vi "log analysis_gps.vi"() -> ()   [LabVIEW 2018] (continued)
status\t114.221582\t125.488390\t7.927600\t-0.997618\t-0.087714\t0.790594\t0.306000\t-0.022000\n\t\n15:12:16.9\tlog_raw\tgps_raw\t\tsystem status\tnormal 2 28.000000 0 0\trobot status\t114.369285\t125.472789\t7.927800\t-0.675524\t-0.152643\t0.044977\t0.313000\t0.000000\n\t\n15:12:17.4\tlog_raw\tgps_raw\t\tsystem status\tnormal 2 28.100000 0 0\trobot status\t114.509051\t125.458503\t7.927000\t-0.401404\t-0.017931\t-0.437891\t0.274000\t-0.037000\n\t\n15:12:17.9\tlog_raw\tgps_raw\t\tsystem status\tnormal 2 28.200000 0 0\trobot status\t114.650658\t125.444370\t7.924700\t-0.327337\t-0.035716\t-0.663327\t0.335000\t0.061000\n\t\n15:12:18.4\tlog_raw\tgps_raw\t\tsystem status\tnormal 2 28.200000 0 0\trobot status\t114.786676\t125.428978\t7.924000\t-0.306443\t0.009430\t-0.778391\t0.296000\t0.002000\n\t\n15:12:18.9\tlog_raw\tgps_raw\t\tsystem status\tnormal 2 28.200000 0 0\trobot status\t114.917132\t125.412522\t7.923700\t-0.381803\t-0.145453\t-0.928746\t0.292000\t0.032000\n\t\n15:12:19.4\tlog_raw\tgps_raw\t#INSPVAXA,USB3,0,47.5,FINESTEERING,2107,281557.450,02000000,471d,15824;INS_ALIGNMENT_COMPLETE,INS_RTKFIXED,37.37126007127,126.72213399175,7.9228,22.3000,-0.0436,0.2932,0.0085,-0.364989974,-0.412142636,90.870623018,0.4100,0.2787,0.5090,0.1093,0.0914,0.0751,0.1708,0.1703,5.1179,0f000001,0*5c4f0bd9\n\tsystem status\tnormal 2 28.200000 0 0\trobot status\t115.053253\t125.397910\t7.922800\t-0.364990\t-0.412143\t-0.870623\t0.296000\t0.029000\n\t\n15:12:19.9\tlog_raw\tgps_raw\t\tsystem status\tnormal 2 28.200000 0 0\trobot status\t115.206485\t125.383092\t7.922200\t-0.467906\t-0.695573\t-0.896423\t0.313000\t0.011000\n\t\n15:12:20.4\tlog_raw\tgps_raw\t#INSPVAXA,USB3,0,46.0,FINESTEERING,2107,281558.450,02000000,471d,15824;INS_ALIGNMENT_COMPLETE,INS_RTKFIXED,37.37125980811,126.72213741354,7.9201,22.3000,-0.0396,0.2827,0.0144,-0.665732137,-0.749833579,90.834139291,0.4087,0.2784,0.5089,0.1102,0.0917,0.0750,0.1706,0.1703,5.1108,0f000001,0*c48606ec\n\tsystem status\tnormal 2 28.200000 0 0\trobot status\t115.356349\t125.368699\t7.920100\t-0.665732\t-0.749834\t-0.834139\t0.304000\t0.025000\n\t\n15:12:20.9\tlog_raw\tgps_raw\t#INSPVAXA,USB3,0,46.0,FINESTEERING,2107,281558.950,02000000,471d,15824;INS_ALIGNMENT_COMPLETE,INS_RTKFIXED,37.37125968631,126.72213896635,7.9182,22.3000,-0.0389,0.2938,0.0155,-0.920394419,-0.718289974,90.450245046,0.4087,0.2784,0.5089,0.1102,0.0917,0.0750,0.1706,0.1703,5.1108,0f000001,0*246e9289\n\tsystem status\tnormal 2 28.100000 0 0\trobot status\t115.493895\t125.355179\t7.918200\t-0.920394\t-0.718290\t-0.450245\t0.249000\t0.114000\n\t\n15:12:21.4\tlog_raw\tgps_raw\t\tsystem status\tnormal 2 28.000000 0 0\trobot status\t115.630698\t125.346330\t7.917200\t-1.162131\t-0.468007\t0.253588\t0.446000\t-0.179000\n\t\n15:12:21.9\tlog_raw\tgps_raw\t\tsystem status\tnormal 2 27.800000 0 0\trobot status\t115.765858\t125.337595\t7.917100\t-1.166059\t-0.209955\t1.295503\t0.319000\t0.012000\n\t\n15:12:22.4\tlog_raw\tgps_raw\t\tsystem status\tnormal 2 27.900000 0 0\trobot status\t115.901706\t125.332414\t7.918000\t-1.105135\t-0.074497\t2.615411\t0.302000\t0.044000\n\t\n15:12:22.9\tlog_raw\tgps_raw\t\tsystem status\tnormal 2 27.800000 0 0\trobot status\t116.038405\t125.330658\t7.919000\t-1.227928\t0.059274\t3.935949\t0.290000\t0.054000\n\t\n15:12:23.4\tlog_raw\tgps_raw\t\tsystem status\tnormal 2 27.800000 0 0\trobot status\t116.176515\t125.336559\t7.920100\t-1.592116\t0.311870\t5.113002\t0.303000\t0.035000\n\t\n15:12:23.9\tlog_raw\tgps_raw\t\tsystem status\tnormal 2 27.900000 0 0\trobot status\t116.315239\t125.343681\t7.923900\t-1.641729\t0.301308\t6.150827\t0.304000\t0.038000\n\t\n15:12:24.4\tlog_raw\tgps_raw\t\tsystem status\tnormal 2 27.900000 0 0\trobot status\t116.455707\t125.354228\t7.925400\t-1.548111\t0.138625\t6.918070\t0.290000\t0.040000\n\t\n15:12:24.9\tlog_raw\tgps_raw\t\tsystem status\tnormal 2 28.000000 0 0\trobot status\t116.600236\t125.367270\t7.927000\t-1.578539\t-0.051102\t7.497431\t0.293000\t0.033000\n\t\n15:12:25.4\tlog_raw\tgps_raw\t\tsystem status\tnormal 2 28.100000 0 0\trobot status\t116.741361\t125.382496\t7.928200\t-1.712113\t-0.033243\t7.732061\t0.302000\t0.000000\n\t\n15:12:25.9\tlog_raw\tgps_raw\t\tsystem status\tnormal 2 28.100000 0 0\trobot status\t116.883583\t125.398503\t7.929100\t-1.939151\t-0.176263\t7.869611\t0.273000\t0.043000\n\t\n15:12:26.4\tlog_raw\tgps_raw\t\tsystem status\tnormal 2 28.200000 0 0\trobot status\t117.028703\t125.414022\t7.929100\t-2.090861\t-0.326492\t7.769708\t0.280000\t0.022000\n\t\n15:12:26.9\tlog_raw\tgps_raw\t\tsystem status\tnormal 2 28.200000 0 0\trobot status\t117.168081\t125.427820\t7.929300\t-2.230499\t-0.413156\t7.644957\t0.298000\t-0.014000\n\t\n15:12:27.4\tlog_raw\tgps_raw\t\tsystem status\tnormal 2 28.200000 0 0\trobot status\t117.306809\t125.442252\t7.930200\t-2.373589\t-0.461391\t7.481825\t0.295000\t-0.036000\n\t\n15:12:27.9\tlog_raw\tgps_raw\t\tsystem status\tnormal 2 28.200000 0 0\trobot status\t117.442588\t125.456064\t7.931900\t-2.514697\t-0.426521\t7.291406\t0.299000\t-0.028000\n\t\n15:12:28.4\tlog_raw\tgps_raw\t\tsystem status\tnormal 2 28.200000 0 0\trobot status\t117.591226\t125.472797\t7.933100\t-2.624686\t-0.295369\t7.089087\t0.297000\t-0.034000\n\t\n15:12:28.9\tlog_raw\tgps_raw\t\tsystem status\tnormal 2 28.200000 0 0\trobot status\t117.743086\t125.488259\t7.934500\t-2.636548\t-0.114819\t6.764470\t0.314000\t-0.013000\n\t\n15:12:29.4\tlog_raw\tgps_raw\t\tsystem status\tnormal 2 28.100000 0 0\trobot status\t117.889876\t125.502021\t7.936500\t-2.818592\t0.030507\t6.232513\t0.329000\t0.006000\n\t\n15:12:29.9\tlog_raw\tgps_raw\t\tsystem status\tnormal 2 28.100000 0 0\trobot status\t118.036258\t125.513145\t7.939400\t-2.805518\t0.155514\t5.496014\t0.331000\t0.001000\n\t\n15:12:30.4\tlog_raw\tgps_raw\t\tsystem status\tnormal 2 28.000000 0 0\trobot status\t118.182757\t125.521347\t7.941500\t-2.864503\t0.225150\t4.530961\t0.274000\t-0.073000\n\t\n15:12:30.9\tlog_raw\tgps_raw\t\tsystem status\tnormal 2 28.000000 0 0\trobot status\t118.328420\t125.525812\t7.943400\t-2.836041\t0.133807\t3.377906\t0.346000\t0.034000\n\t\n15:12:31.4\tlog_raw\tgps_raw\t\tsystem status\tnormal 2 28.000000 0 0\trobot status\t118.477303\t125.526010\t7.944100\t-2.591603\t-0.053217\t2.197763\t0.321000\t0.003000\n\t\n15:12:31.9\tlog_raw\tgps_raw\t\tsystem status\tnormal 2 28.000000 0 0\trobot status\t118.625287\t125.523387\t7.945600\t-2.386968\t-0.298776\t1.066511\t0.307000\t-0.023000\n\t\n15:12:32.4\tlog_raw\tgps_raw\t\tsystem status\tnormal 2 28.000000 0 0\trobot status\t118.774658\t125.518337\t7.947800\t-2.206603\t-0.548381\t-0.008470\t0.298000\t-0.023000\n\t\n15:12:32.9\tlog_raw\tgps_raw\t\tsystem status\tnormal 2 28.000000 0 0\trobot status\t118.921009\t125.512839\t7.950800\t-2.307420\t-0.567833\t-0.931552\t0.270000\t-0.065000\n\t\n15:12:33.4\tlog_raw\tgps_raw\t\tsystem status\tnormal 2 28.100000 0 0\trobot status\t119.066666\t125.504844\t7.951000\t-2.313842\t-0.584866\t-1.577300\t0.333000\t0.029000\n\t\n15:12:33.9\tlog_raw\tgps_raw\t\tsystem status\tnormal 2 28.100000 0 0\trobot status\t119.210312\t125.494692\t7.951000\t-2.168611\t-0.499585\t-1.946386\t0.457000\t0.245000\n\t\n15:12:34.4\tlog_raw\tgps_raw\t\tsystem status\tnormal 2 28.200000 0 0\trobot status\t119.354380\t125.482079\t7.951900\t-2.009888\t-0.430352\t-2.250968\t0.348000\t0.076000\n\t\n15:12:34.9\tlog_raw\tgps_raw\t\tsystem status\tnormal 2 28.200000 0 0\trobot status\t119.492909\t125.469474\t7.954700\t-1.965925\t-0.157568\t-2.482807\t0.285000\t-0.004000\n\t\n15:12:35.4\tlog_raw\tgps_raw\t\tsystem status\tnormal 2 28.200000 0 0\trobot status\t119.630126\t125.456372\t7.956500\t-1.882753\t0.008838\t-2.666533\t0.300000\t0.016000\n\t\n15:12:35.9\tlog_raw\tgps_raw\t\tsystem status\tnormal 2 28.200000 0 0\trobot status\t119.763943\t125.442716\t7.958800\t-1.738197\t0.188816\t-2.820552\t0.297000\t0.013000\n\t\n15:12:36.5\tlog_raw\tgps_raw\t\tsystem status\tnormal 2 28.200000 0 0\trobot status\t119.902164\t125.427889\t7.960300\t-1.597063\t0.344693\t-2.879224\t0.300000\t0.014000\n\t\n15:12:37.0\tlog_raw\tgps_raw\t\tsystem status\tnormal 2 28.200000 0 0\trobot status\t120.045429\t125.413001\t7.962300\t-1.509715\t0.381966\t-2.910897\t0.304000\t0.024000\n\t\n15:12:37.5\tlog_raw\tgps_raw\t\tsystem status\tnormal 2 28.200000 0 0\trobot status\t120.194407\t125.398465\t7.963800\t-1.498522\t0.411743\t-2.852737\t0.305000\t0.014000\n\t\n15:12:38.0\tlog_raw\tgps_raw\t\tsystem status\tnormal 2 28.200000 0 0\trobot status\t120.343490\t125.382080\t7.966000\t-1.287003\t0.328447\t-2.767215\t0.385000\t-0.091000\n\t\n15:12:38.5\tlog_raw\tgps_raw\t\tsystem status\tnormal 2 28.100000 0 0\trobot status\t120.485030\t125.365356\t7.967200\t-1.104160\t0.161834\t-2.356447\t0.268000\t0.066000\n\t\n15:12:39.0\tlog_raw\tgps_raw\t\tsystem status\tnormal 2 28.000000 0 0\trobot status\t120.628511\t125.350613\t7.968100\t-1.128954\t-0.000573\t-1.759684\t0.343000\t-0.041000\n\t\n15:12:39.5\tlog_raw\tgps_raw\t\tsystem status\tnormal 2 28.000000 0 0\trobot status\t120.770142\t125.337474\t7.968500\t-1.185835\t-0.189580\t-0.843939\t0.284000\t0.061000\n\t\n15:12:40.0\tlog_raw\tgps_raw\t\tsystem status\tnormal 2 27.900000 0 0\trobot status\t120.910677\t125.325028\t7.970200\t-1.109067\t-0.244345\t0.105658\t0.239000\t0.130000\n\t\n15:12:40.5\tlog_raw\tgps_raw\t\tsystem status\tnormal 2 27.900000 0 0\trobot status\t121.053149\t125.315896\t7.971400\t-1.028445\t-0.286591\t1.145120\t0.290000\t0.037000\n\t\n15:12:41.0\tlog_raw\tgps_raw\t\tsystem status\tnormal 2 27.900000 0 0\trobot status\t121.194941\t125.310241\t7.971600\t-1.057766\t-0.377621\t2.167851\t0.306000\t0.032000\n\t\n15:12:41.5\tlog_raw\tgps_raw\t\tsystem status\tnormal 2 27.900000 0 0\trobot status\t121.336529\t125.307382\t7.970900\t-1.082553\t-0.380854\t2.986271\t0.309000\t0.014000\n\t\n15:12:42.0\tlog_raw\tgps_raw\t\tsystem status\tnormal 2 28.000000 0 0\trobot status\t121.476056\t125.305407\t7.970800\t-1.037994\t-0.335717\t3.686672\t0.316000\t-0.003000\n\t\n15:12:42.5\tlog_raw\tgps_raw\t\tsystem status\tnormal 2 28.100000 0 0\trobot status\t121.618655\t125.305174\t7.968300\t-0.855579\t-0.321584\t4.290336\t0.294000\t0.018000\n\t\n15:12:43.0\tlog_raw\tgps_raw\t\tsystem status\tnormal 2 28.100000 0 0\trobot status\t121.761079\t125.306348\t7.965900\t-0.820878\t-0.229531\t4.658904\t0.359000\t-0.087000\n\t\n15:12:43.5\tlog_raw\tgps_raw\t\tsystem status\tnormal 2 28.100000 0 0\trobot status\t121.904568\t125.307348\t7.964700\t-0.804642\t-0.120822\t4.991098\t0.239000\t0.092000\n\t\n15:12:44.0\tlog_raw\tgps_raw\t#INSPVAXA,USB3,0,48.5,FINESTEERING,2107,281582.000,02000000,471d,15824;INS_ALIGNMENT_COMPLETE,INS_RTKFIXED,37.37125926697,126.72221314243,7.9638,22.3000,0.0065,0.2832,0.0220,-0.844956483,-0.026158862,84.896486231,0.4081,0.2757,0.5033,0.1092,0.0895,0.0749,0.1683,0.1693,5.0877,0f000001,0*999c2cb4\n\tsystem status\tnormal 2 28.100000 0 0\trobot status\t122.064290\t125.308546\t7.963800\t-0.844956\t-0.026159\t5.103514\t0.245000\t0.071000\n\t\n15:12:44.5\tlog_raw\tgps_raw\t\tsystem status\tnormal 2 28.200000 0 0\trobot status\t122.196254\t125.311549\t7.961600\t-0.819027\t-0.077937\t5.145160\t0.253000\t0.067000\n\t\n15:12:45.0\tlog_raw\tgps_raw\t\tsystem status\tnormal 2 28.200000 0 0\trobot status\t122.339384\t125.314418\t7.961000\t-0.796553\t-0.063929\t5.057289\t0.299000\t0.003000\n\t\n15:12:45.5\tlog_raw\tgps_raw\t\tsystem status\tnormal 2 28.200000 0 0\trobot status\t122.480026\t125.316859\t7.961500\t-0.623838\t-0.052585\t4.997421\t0.300000\t-0.015000\n\t\n15:12:46.0\tlog_raw\tgps_raw\t\tsystem status\tnormal 2 28.200000 0 0\trobot status\t122.625961\t125.319868\t7.962800\t-0.512158\t0.039063\t4.891970\t0.298000\t-0.014000\n\t\n15:12:46.5\tlog_raw\tgps_raw\t\tsystem status\tnormal 2 28.200000 0 0\trobot status\t122.765847\t125.322078\t7.963900\t-0.593182\t0.086025\t4.816919\t0.298000\t-0.015000\n\t\n15:12:47.0\tlog_raw\tgps_raw\t#INSPVAXA,USB3,0,45.5,FINESTEERING,2107,281585.000,02000000,471d,15824;INS_ALIGNMENT_COMPLETE,INS_RTKFIXED,37.37125940272,126.72222284495,7.9649,22.3000,-0.0095,0.2865,0.0182,-0.747268326,0.234159981,85.317572401,0.4076,0.2752,0.5032,0.1094,0.0898,0.0748,0.1683,0.1693,5.0921,0f000001,0*05cc0da4\n\tsystem status\tnormal 2 28.200000 0 0\trobot status\t122.923724\t125.323599\t7.964900\t-0.747268\t0.234160\t4.682428\t0.298000\t-0.017000\n\t\n15:12:47.5\tlog_raw\tgps_raw\t#INSPVAXA,USB3,0,49.5,FINESTEERING,2107,281585.500,02000000,471d,15824;INS_ALIGNMENT_COMPLETE,INS_RTKFIXED,37.37125941547,126.72222448778,7.9662,22.3000,-0.0142,0.2884,0.0124,-0.699076432,0.369703687,85.497806859,0.4078,0.2753,0.5032,0.1096,0.0899,0.0748,0.1684,0.1693,5.0937,0f000001,0*7e52f1b7\n\tsystem status\tnormal 2 28.200000 0 0\trobot status\t123.069243\t125.325012\t7.966200\t-0.699076\t0.369704\t4.502193\t0.299000\t-0.019000\n\t\n15:12:48.0\tlog_raw\tgps_raw\t\tsystem status\tnormal 2 28.200000 0 0\trobot status\t123.201866\t125.324412\t7.968200\t-0.615056\t0.373117\t4.351068\t0.301000\t-0.020000\n\t\n15:12:48.5\tlog_raw\tgps_raw\t#INSPVAXA,USB3,0,49.5,FINESTEERING,2107,281586.500,02000000,471d,15824;INS_ALIGNMENT_COMPLETE,INS_RTKFIXED,37.37125940571,126.72222789541,7.9680,22.3000,0.0030,0.3079,0.0233,-0.562980027,0.263238278,85.915106652,0.4081,0.2752,0.5032,0.1097,0.0899,0.0748,0.1684,0.1692,5.0953,0f000001,0*7d04a5bf\n\tsystem status\tnormal 2 28.200000 0 0\trobot status\t123.371085\t125.323924\t7.968000\t-0.562980\t0.263238\t4.084893\t0.300000\t-0.024000\n\t\n15:12:49.0\tlog_raw\tgps_raw\t#INSPVAXA,USB3,0,49.5,FINESTEERING,2107,281587.000,02000000,471d,15824;INS_ALIGNMENT_COMPLETE,INS_RTKFIXED,37.37125938358,126.72222955995,7.9677,22.3000,-0.0088,0.3126,0.0171,-0.528697229,0.195556365,86.199096589,0.4081,0.2752,0.5032,0.1097,0.0899,0.0748,0.1684,0.1692,5.0953,0f000001,0*98856aba\n\tsystem status\tnormal 2 28.200000 0 0\trobot status\t123.518527\t125.321466\t7.967700\t-0.528697\t0.195556\t3.800903\t0.299000\t-0.026000\n\t\n15:12:49.5\tlog_raw\tgps_raw\t#INSPVAXA,USB3,0,47.0,FINESTEERING,2107,281587.500,02000000,471d,15824;INS_ALIGNMENT_COMPLETE,INS_RTKFIXED,37.37125935739,126.72223128487,7.9668,22.3000,-0.0030,0.3090,0.0190,-0.470354496,0.052583887,86.493869068,0.4079,0.2752,0.5030,0.1098,0.0899,0.0747,0.1684,0.1690,5.0969,0f000001,0*c1a2a853\n\tsystem status\tnormal 2 28.200000 0 0\trobot status\t123.671318\t125.318557\t7.966800\t-0.470354\t0.052584\t3.506131\t0.303000\t-0.014000\n\t\n15:12:50.0\tlog_raw\tgps_raw\t\tsystem status\tnormal 2 28.200000 0 0\trobot status\t123.806018\t125.313632\t7.966100\t-0.342863\t-0.216734\t3.135832\t0.303000\t-0.013000\n\t\n15:12:50.5\tlog_raw\tgps_raw\t\tsystem status\tnormal 2 28.100000 0 0\trobot status\t123.954300\t125.308376\t7.964100\t-0.347670\t-0.390101\t2.769340\t0.275000\t-0.061000\n\t\n15:12:51.0\tlog_raw\tgps_raw\t\tsystem status\tnormal 2 28.200000 0 0\trobot status\t124.102892\t125.299937\t7.962000\t-0.229727\t-0.448052\t2.357435\t0.281000\t-0.049000\n\t\n15:12:51.5\tlog_raw\tgps_raw\t\tsystem status\tnormal 2 28.100000 0 0\trobot status\t124.248033\t125.291272\t7.959900\t-0.042738\t-0.400002\t1.929677\t0.287000\t-0.030000\n\t\n15:12:52.0\tlog_raw\tgps_raw\t\tsystem status\tnormal 2 28.100000 0 0\trobot status\t124.392663\t125.281272\t7.957200\t-0.008101\t-0.177855\t1.517386\t0.250000\t-0.086000\n\t\n15:12:52.5\tlog_raw\tgps_raw\t#INSPVAXA,USB3,0,45.5,FINESTEERING,2107,281590.500,02000000,471d,15824;INS_ALIGNMENT_COMPLETE,INS_RTKFIXED,37.37125890881,126.72224121064,7.9541,22.3000,-0.0384,0.3088,0.0049,0.158198742,0.001802096,88.889148367,0.4071,0.2753,0.5028,0.1097,0.0897,0.0747,0.1683,0.1686,5.0995,0f000001,0*955ddbd0\n\tsystem status\tnormal 2 28.100000 0 0\trobot status\t124.550526\t125.268759\t7.954100\t0.158199\t0.001802\t1.110852\t0.283000\t-0.049000\n\t\n15:12:53.0\tlog_raw\tgps_raw\t#INSPVAXA,USB3,0,45.5,FINESTEERING,2107,281591.000,02000000,471d,15824;INS_ALIGNMENT_COMPLETE,INS_RTKFIXED,37.37125878805,126.72224284394,7.9517,22.3000,-0.0402,0.3180,0.0042,0.353980649,0.071732685,89.195409994,0.4071,0.2753,0.5028,0.1097,0.0897,0.0747,0.1683,0.1686,5.0995,0f000001,0*1c59d57f\n\tsystem status\tnormal 2 28.200000 0 0\trobot status\t124.695201\t125.255354\t7.951700\t0.353981\t0.071733\t0.804590\t0.299000\t-0.018000\n\t\n15:12:53.5\tlog_raw\tgps_raw\t#INSPVAXA,USB3,0,48.0,FINESTEERING,2107,281591.500,02000000,471d,15824;INS_ALIGNMENT_COMPLETE,INS_RTKFIXED,37.37125869638,126.72224442366,7.9492,22.3000,-0.0439,0.3158,0.0021,0.440194436,0.083978033,89.508465675,0.4069,0.2753,0.5025,0.1096,0.0897,0.0747,0.1683,0.1685,5.0994,0f000001,0*cd52a6fa\n\tsystem status\tnormal 2 28.200000 0 0\trobot status\t124.835130\t125.245178\t7.949200\t0.440194\t0.083978\t0.491534\t0.340000\t0.054000\n\t\n15:12:54.0\tlog_raw\tgps_raw\t\tsystem status\tnormal 2 28.200000 0 0\trobot status\t124.962153\t125.235317\t7.947900\t0.376018\t0.054716\t0.341333\t0.278000\t-0.019000\n\t\n15:12:54.5\tlog_raw\tgps_raw\t#INSPVAXA,USB3,0,49.0,FINESTEERING,2107,281592.500,02000000,471d,15824;INS_ALIGNMENT_COMPLETE,INS_RTKFIXED,37.37125852305,126.72224758487,7.9467,22.3000,-0.0419,0.2989,0.0081,0.241164768,-0.091182939,89.866254951,0.4067,0.2753,0.5023,0.1093,0.0896,0.0746,0.1683,0.1684,5.0986,0f000001,0*7410d7bd\n\tsystem status\tnormal 2 28.200000 0 0\trobot status\t125.115145\t125.225937\t7.946700\t0.241165\t-0.091183\t0.133745\t0.298000\t0.002000\n\t\n15:12:55.0\tlog_raw\tgps_raw\t#INSPVAXA,USB3,0,49.0,FINESTEERING,2107,281593.000,02000000,471d,15824;INS_ALIGNMENT_COMPLETE,INS_RTKFIXED,37.37125843294,126.72224909789,7.9463,22.3000,-0.0494,0.2967,0.0111,0.084019586,0.037300325,90.030415864,0.4067,0.2753,0.5023,0.1093,0.0896,0.0746,0.1683,0.1684,5.0986,0f000001,0*0c6e6e15\n\tsystem status\tnormal 2 28.200000 0 0\trobot status\t125.249166\t125.215934\t7.946300\t0.084020\t0.037300\t-0.030416\t0.297000\t0.011000\n\t\n15:12:55.5\tlog_raw\tgps_raw\t#INSPVAXA,USB3,0,47.0,FINESTEERING,2107,281593.500,02000000,471d,15824;INS_ALIGNMENT_COMPLETE,INS_RTKFIXED,37.37125834817,126.72225064621,7.9448,22.3000,-0.0530,0.2881,0.0083,-0.027403360,0.078247142,90.176817811,0.4066,0.2752,0.5020,0.1093,0.0894,0.0746,0.1682,0.1684,5.0980,0f000001,0*f779539b\n\tsystem status\tnormal 2 28.200000 0 0\trobot status\t125.386314\t125.206524\t7.944800\t-0.027403\t0.078247\t-0.176818\t0.300000\t0.011000\n\t\n15:12:56.0\tlog_raw\tgps_raw\t\tsystem status\tnormal 2 28.200000 0 0\trobot status\t125.511915\t125.196305\t7.943100\t-0.041322\t0.071389\t-0.260501\t0.304000\t0.011000\n\t\n15:12:56.5\tlog_raw\tgps_raw\t#INSPVAXA,USB3,0,49.0,FINESTEERING,2107,281594.500,02000000,471d,15824;INS_ALIGNMENT_COMPLETE,INS_RTKFIXED,37.37125815716,126.72225388561,7.9395,22.3000,-0.0550,0.3023,0.0057,-0.022782572,-0.170277850,90.320435048,0.4065,0.2750,0.5018,0.1093,0.0894,0.0746,0.1682,0.1684,5.0981,0f000001,0*f8af8c2b\n\tsystem status\tnormal 2 28.200000 0 0\trobot status\t125.673254\t125.185320\t7.939500\t-0.022783\t-0.170278\t-0.320435\t0.296000\t0.011000\n\t\n15:12:57.0\tlog_raw\tgps_raw\t#INSPVAXA,USB3,0,49.0,FINESTEERING,2107,281595.000,02000000,471d,15824;INS_ALIGNMENT_COMPLETE,INS_RTKFIXED,37.37125806903,126.72225552746,7.9370,22.3000,-0.0572,0.3021,0.0033,-0.060546798,-0.376099237,90.424899163,0.4065,0.2750,0.5018,0.1093,0.0894,0.0746,0.1682,0.1684,5.0981,0f000001,0*15f57f01\n\tsystem status\tnormal 2 28.200000 0 0\trobot status\t125.818687\t125.175537\t7.937000\t-0.060547\t-0.376099\t-0.424899\t0.297000\t0.019000\n\t\n15:12:57.5\tlog_raw\tgps_raw\t\tsystem status\tnormal 2 28.200000 0 0\trobot status\t125.947677\t125.168074\t7.936100\t-0.265856\t-0.446178\t-0.462441\t0.244000\t0.100000\n\t\n15:12:58.0\tlog_raw\tgps_raw\t#INSPVAXA,USB3,0,49.0,FINESTEERING,2107,281596.000,02000000,471d,15824;INS_ALIGNMENT_COMPLETE,INS_RTKFIXED,37.37125790124,126.72225886435,7.9333,22.3000,-0.0466,0.2890,0.0127,-0.410308498,-0.648762908,90.450935074,0.4065,0.2747,0.5016,0.1095,0.0895,0.0746,0.1681,0.1684,5.0986,0f000001,0*6915a645\n\tsystem status\tnormal 2 28.200000 0 0\trobot status\t126.114263\t125.156910\t7.933300\t-0.410308\t-0.648763\t-0.450935\t0.260000\t0.063000\n\t\n15:12:58.5\tlog_raw\tgps_raw\t#INSPVAXA,USB3,0,49.5,FINESTEERING,2107,281596.500,02000000,471d,15824;INS_ALIGNMENT_COMPLETE,INS_RTKFIXED,37.37125781382,126.72226046483,7.9311,22.3000,-0.0418,0.2833,0.0090,-0.435085374,-0.543120061,90.230742577,0.4063,0.2745,0.5015,0.1095,0.0898,0.0746,0.1681,0.1684,5.0990,0f000001,0*49551541\n\tsystem status\tnormal 2 28.100000 0 0\trobot status\t126.256031\t125.147206\t7.931100\t-0.435085\t-0.543120\t-0.230743\t0.372000\t-0.097000\n\t\n15:12:59.0\tlog_raw\tgps_raw\t#INSPVAXA,USB3,0,49.5,FINESTEERING,2107,281597.000,02000000,471d,15824;INS_ALIGNMENT_COMPLETE,INS_RTKFIXED,37.37125771210,126.72226205669,7.9296,22.3000,-0.0419,0.3034,0.0146,-0.176475968,-0.465211146,89.900752535,0.4063,0.2745,0.5015,0.1095,0.0898,0.0746,0.1681,0.1684,5.0990,0f000001,0*aa558b24\n\tsystem status\tnormal 2 28.100000 0 0\trobot status\t126.397035\t125.135914\t7.929600\t-0.176476\t-0.465211\t0.099247\t0.292000\t0.036000\n\t\n15:12:59.5\tlog_raw\tgps_raw\t#INSPVAXA,USB3,0,50.0,FINESTEERING,2107,281597.500,02000000,471d,15824;INS_ALIGNMENT_COMPLETE,INS_RTKFIXED,37.37125762620,126.72226364430,7.9270,22.3000,-0.0431,0.2944,0.0123,-0.034850827,-0.383453655,89.494102450,0.4062,0.2742,0.5014,0.1094,0.0896,0.0746,0.1680,0.1684,5.0989,0f000001,0*eb33c8cb\n\tsystem status\tnormal 2 28.100000 0 0\trobot status\t126.537663\t125.126379\t7.927000\t-0.034851\t-0.383454\t0.505898\t0.347000\t-0.054000\n\t\n15:13:00.0\tlog_raw\tgps_raw\t#INSPVAXA,USB3,0,50.0,FINESTEERING,2107,281598.000,02000000,471d,15824;INS_ALIGNMENT_COMPLETE,INS_RTKFIXED,37.37125755430,126.72226525077,7.9232,22.3000,-0.0288,0.2974,0.0131,0.018056318,-0.346106265,89.006732847,0.4062,0.2742,0.5014,0.1094,0.0896,0.0746,0.1680,0.1684,5.0989,0f000001,0*7f8cff1a\n\tsystem status\tnormal 2 28.100000 0 0\trobot status\t126.679962\t125.118397\t7.923200\t0.018056\t-0.346106\t0.993267\t0.336000\t-0.025000\n\t\n15:13:00.5\tlog_raw\tgps_raw\t#INSPVAXA,USB3,0,47.5,FINESTEERING,2107,281598.500,02000000,471d,15824;INS_ALIGNMENT_COMPLETE,INS_RTKFIXED,37.37125752692,126.72226686003,7.9200,22.3000,-0.0297,0.2922,-0.0044,-0.122753848,-0.350679185,88.582247328,0.4061,0.2743,0.5013,0.1093,0.0895,0.0746,0.1680,0.1684,5.0986,0f000001,0*76a956e7\n\tsystem status\tnormal 2 28.100000 0 0\trobot status\t126.822507\t125.115356\t7.920000\t-0.122754\t-0.350679\t1.417753\t0.184000\t0.200000\n\t\n15:13:01.0\tlog_raw\tgps_raw\t#INSPVAXA,USB3,0,47.5,FINESTEERING,2107,281599.000,02000000,471d,15824;INS_ALIGNMENT_COMPLETE,INS_RTKFIXED,37.37125750157,126.72226846220,7.9172,22.3000,-0.0394,0.2975,0.0004,-0.262738431,-0.259927736,88.093141362,0.4061,0.2743,0.5013,0.1093,0.0895,0.0746,0.1680,0.1684,5.0986,0f000001,0*5a405d12\n\tsystem status\tnormal 2 28.100000 0 0\trobot status\t126.964425\t125.112540\t7.917200\t-0.262738\t-0.259928\t1.906859\t0.182000\t0.194000\n\t\n15:13:01.5\tlog_raw\tgps_raw\t#INSPVAXA,USB3,0,47.5,FINESTEERING,2107,281599.500,02000000,471d,15824;INS_ALIGNMENT_COMPLETE,INS_RTKFIXED,37.37125749812,126.72227005344,7.9138,22.3000,-0.0467,0.2803,-0.0089,-0.269229202,-0.225074216,87.528625301,0.4063,0.2743,0.5013,0.1092,0.0896,0.0746,0.1679,0.1685,5.0987,0f000001,0*0f923b8c\n\tsystem status\tnormal 2 28.000000 0 0\trobot status\t127.105374\t125.112155\t7.913800\t-0.269229\t-0.225074\t2.471375\t0.348000\t-0.048000\n\t\n15:13:02.0\tlog_raw\tgps_raw\t#INSPVAXA,USB3,0,47.5,FINESTEERING,2107,281600.000,02000000,471d,15824;INS_ALIGNMENT_COMPLETE,INS_RTKFIXED,37.37125749625,126.72227167040,7.9096,22.3000,-0.0440,0.2738,-0.0170,-0.124807872,-0.330803531,87.082207442,0.4063,0.2743,0.5013,0.1092,0.0896,0.0746,0.1679,0.1685,5.0987,0f000001,0*844dad1a\n\tsystem status\tnormal 2 28.000000 0 0\trobot status\t127.248602\t125.111946\t7.909600\t-0.124808\t-0.330804\t2.917793\t0.282000\t0.040000\n\t\n15:13:02.5\tlog_raw\tgps_raw\t#DUALANTENNAHEADINGA,USB3,0,49.5,FINESTEERING,2107,281600.500,02000000,d426,15824;SOL_COMPUTED,NARROW_FLOAT,-1.000000000,72.063247681,-40.725646973,0.0,273.105743408,180.000000000,\"631T\",22,8,8,8,04,00,20,23*8da2d13b\n\tsystem status\tnormal 2 28.100000 0 0\trobot status\t127.390966\t125.113507\t7.906200\t-0.209027\t-0.281844\t3.127823\t0.231000\t0.117000\n\t\n15:13:03.0\tlog_raw\tgps_raw\t#INSPVAXA,USB3,0,49.5,FINESTEERING,2107,281601.000,02000000,471d,15824;INS_ALIGNMENT_COMPLETE,INS_RTKFIXED,37.37125751795,126.72227489272,7.9035,22.3000,-0.0358,0.2988,-0.0067,-0.198567071,-0.277392805,86.699743211,0.4065,0.2744,0.5014,0.1092,0.0895,0.0746,0.1679,0.1685,5.0988,0f000001,0*2cadf3ab\n\tsystem status\tnormal 2 28.100000 0 0\trobot status\t127.534030\t125.114350\t7.903500\t-0.198567\t-0.277393\t3.300257\t0.353000\t-0.073000\n\t\n15:13:03.5\tlog_raw\tgps_raw\t#INSPVAXA,USB3,0,48.0,FINESTEERING,2107,281601.500,02000000,471d,15824;INS_ALIGNMENT_COMPLETE,INS_RTKFIXED,37.37125754133,126.72227651684,7.9018,22.3000,-0.0303,0.2880,-0.0022,-0.260652081,-0.486725638,86.696539818,0.4068,0.2744,0.5014,0.1092,0.0895,0.0746,0.1679,0.1685,5.0994,0f000001,0*3e737448\n\tsystem status\tnormal 2 28.100000 0 0\trobot status\t127.677892\t125.116942\t7.901800\t-0.260652\t-0.486726\t3.303460\t0.240000\t0.088000\n\t\n15:13:04.0\tlog_raw\tgps_raw\t#INSPVAXA,USB3,0,48.0,FINESTEERING,2107,281602.000,02000000,471d,15824;INS_ALIGNMENT_COMPLETE,INS_RTKFIXED,37.37125756266,126.72227812513,7.9001,22.3000,-0.0263,0.2865,-0.0045,-0.342075300,-0.515152561,86.801185345,0.4068,0.2744,0.5014,0.1092,0.0895,0.0746,0.1679,0.1685,5.0994,0f000001,0*64049b1c\n\tsystem status\tnormal 2 28.200000 0 0\trobot status\t127.820351\t125.119307\t7.900100\t-0.342075\t-0.515153\t3.198815\t0.328000\t-0.062000\n\t\n15:13:04.5\tlog_raw\tgps_raw\t#INSPVAXA,USB3,0,49.0,FINESTEERING,2107,281602.500,02000000,471d,15824;INS_ALIGNMENT_COMPLETE,INS_RTKFIXED,37.37125758385,126.72227971181,7.8988,22.3000,-0.0248,0.2942,-0.0059,-0.465449953,-0.482180985,86.903233906,0.4069,0.2744,0.5013,0.1092,0.0896,0.0746,0.1678,0.1685,5.1000,0f000001,0*df1bf2df\n\tsystem status\tnormal 2 28.200000 0 0\trobot status\t127.960897\t125.121657\t7.898800\t-0.465450\t-0.482181\t3.096766\t0.295000\t-0.011000\n\t\n15:13:05.0\tlog_raw\tgps_raw\t#INSPVAXA,USB3,0,49.0,FINESTEERING,2107,281603.000,02000000,471d,15824;INS_ALIGNMENT_COMPLETE,INS_RTKFIXED,37.37125760896,126.72228133197,7.8974,22.3000,-0.0248,0.2888,-0.0003,-0.623364268,-0.535478966,87.043420803,0.4069,0.2744,0.5013,0.1092,0.0896,0.0746,0.1678,0.1685,5.1000,0f000001,0*b0d9f6c7\n\tsystem status\tnormal 2 28.200000 0 0\trobot status\t128.104408\t125.124442\t7.897400\t-0.623364\t-0.535479\t2.956579\t0.295000\t-0.018000\n\t\n15:13:05.5\tlog_raw\tgps_raw\t#INSPVAXA,USB3,0,49.5,FINESTEERING,2107,281603.500,02000000,471d,15824;INS_ALIGNMENT_COMPLETE,INS_RTKFIXED,37.37125762014,126.72228294521,7.8952,22.3000,-0.0259,0.2842,0.0002,-0.657593864,-0.460325437,87.196665885,0.4072,0.2744,0.5014,0.1092,0.0897,0.0746,0.1678,0.1686,5.1007,0f000001,0*32d6fd63\n\tsystem status\tnormal 2 28.200000 0 0\trobot status\t128.247306\t125.125680\t7.895200\t-0.657594\t-0.460325\t2.803334\t0.301000\t-0.020000\n\t\n15:13:06.0\tlog_raw\tgps_raw\t#INSPVAXA,USB3,0,49.5,FINESTEERING,2107,281604.000,02000000,471d,15824;INS_ALIGNMENT_COMPLETE,INS_RTKFIXED,37.37125761729,126.72228447790,7.8935,22.3000,-0.0300,0.2898,-0.0081,-0.656830012,-0.299740331,87.333790648,0.4072,0.2744,0.5014,0.1092,0.0897,0.0746,0.1678,0.1686,5.1007,0f000001,0*76a7715c\n\tsystem status\tnormal 2 28.200000 0 0\trobot status\t128.383069\t125.125362\t7.893500\t-0.656830\t-0.299740\t2.666209\t0.296000\t-0.018000\n\t\n15:13:06.5\tlog_raw\tgps_raw\t#INSPVAXA,USB3,0,44.5,FINESTEERING,2107,281604.500,02000000,471d,15824;INS_ALIGNMENT_COMPLETE,INS_RTKFIXED,37.37125762223,126.72228607343,7.8940,22.3000,-0.0219,0.2910,-0.0031,-0.589546235,-0.368304883,87.506526746,0.4072,0.2745,0.5015,0.1092,0.0897,0.0746,0.1678,0.1685,5.1010,0f000001,0*388a7a2d\n\tsystem status\tnormal 2 28.200000 0 0\trobot status\t128.524399\t125.125908\t7.894000\t-0.589546\t-0.368305\t2.493473\t0.298000\t-0.019000\n\t\n15:13:07.0\tlog_raw\tgps_raw\t#INSPVAXA,USB3,0,44.5,FINESTEERING,2107,281605.000,02000000,471d,15824;INS_ALIGNMENT_COMPLETE,INS_RTKFIXED,37.37125762402,126.72228771590,7.8945,22.3000,-0.0210,0.3023,-0.0017,-0.565411059,-0.344280902,87.705183727,0.4072,0.2745,0.5015,0.1092,0.0897,0.0746,0.1678,0.1685,5.1010,0f000001,0*43df75d8\n\tsystem status\tnormal 2 28.200000 0 0\trobot status\t128.669886\t125.126104\t7.894500\t-0.565411\t-0.344281\t2.294816\t0.299000\t-0.029000\n\t\n15:13:07.5\tlog_raw\tgps_raw\t#INSPVAXA,USB3,0,49.5,FINESTEERING,2107,281605.500,02000000,471d,15824;INS_ALIGNMENT_COMPLETE,INS_RTKFIXED,37.37125763713,126.72228942548,7.8937,22.3000,-0.0187,0.2984,0.0018,-0.682644637,-0.329022185,87.922528604,0.4076,0.2746,0.5016,0.1093,0.0897,0.0746,0.1678,0.1685,5.1013,0f000001,0*79d36c9f\n\tsystem status\tnormal 2 28.200000 0 0\trobot status\t128.821318\t125.127557\t7.893700\t-0.682645\t-0.329022\t2.077471\t0.299000\t-0.018000\n\t\n15:13:08.0\tlog_raw\tgps_raw\t#INSPVAXA,USB3,0,49.5,FINESTEERING,2107,281606.000,02000000,471d,15824;INS_ALIGNMENT_COMPLETE,INS_RTKFIXED,37.37125764382,126.72229106534,7.8933,22.3000,-0.0223,0.2951,0.0001,-0.712476765,-0.315068530,88.171988719,0.4076,0.2746,0.5016,0.1093,0.0897,0.0746,0.1678,0.1685,5.1013,0f000001,0*a3ebc004\n\tsystem status\tnormal 2 28.200000 0 0\trobot status\t128.966574\t125.128297\t7.893300\t-0.712477\t-0.315069\t1.828011\t0.305000\t-0.017000\n\t\n15:13:08.5\tlog_raw\tgps_raw\t#INSPVAXA,USB3,0,50.0,FINESTEERING,2107,281606.500,02000000,471d,15824;INS_ALIGNMENT_COMPLETE,INS_RTKFIXED,37.37125763803,126.72229270568,7.8917,22.3000,-0.0150,0.3037,-0.0036,-0.690294492,-0.219977588,88.452886392,0.4077,0.2746,0.5015,0.1093,0.0897,0.0746,0.1678,0.1685,5.1018,0f000001,0*e1d1f507\n\tsystem status\tnormal 2 28.200000 0 0\trobot status\t129.111873\t125.127652\t7.891700\t-0.690294\t-0.219978\t1.547114\t0.309000\t-0.019000\n\t\n15:13:09.0\tlog_raw\tgps_raw\t#INSPVAXA,USB3,0,50.0,FINESTEERING,2107,281607.000,02000000,471d,15824;INS_ALIGNMENT_COMPLETE,INS_RTKFIXED,37.37125762815,126.72229434491,7.8899,22.3000,-0.0081,0.2973,0.0070,-0.653085669,-0.059361264,88.754704590,0.4077,0.2746,0.5015,0.1093,0.0897,0.0746,0.1678,0.1685,5.1018,0f000001,0*aec8b341\n\tsystem status\tnormal 2 28.200000 0 0\trobot status\t129.257073\t125.126554\t7.889900\t-0.653086\t-0.059361\t1.245295\t0.355000\t0.062000\n\t\n15:13:09.5\tlog_raw\tgps_raw\t#INSPVAXA,USB3,0,50.5,FINESTEERING,2107,281607.500,02000000,471d,15824;INS_ALIGNMENT_COMPLETE,INS_RTKFIXED,37.37125761017,126.72229595804,7.8881,22.3000,-0.0137,0.2967,-0.0028,-0.749913481,-0.074231806,89.214794289,0.4080,0.2746,0.5014,0.1093,0.0897,0.0746,0.1678,0.1684,5.1022,0f000001,0*37633f72\n\tsystem status\tnormal 2 28.200000 0 0\trobot status\t129.399961\t125.124556\t7.888100\t-0.749913\t-0.074232\t0.785206\t0.369000\t0.076000\n\t\n15:13:10.0\tlog_raw\tgps_raw\t#DUALANTENNAHEADINGA,USB3,0,50.5,FINESTEERING,2107,281608.000,02000000,d426,15824;SOL_COMPUTED,NARROW_FLOAT,-1.000000000,78.494079590,-41.424682617,0.0,180.103469849,180.000000000,\"631T\",21,10,10,8,04,00,20,23*2f530816\n\tsystem status\tnormal 2 28.200000 0 0\trobot status\t129.544107\t125.121422\t7.886100\t-0.808999\t-0.274037\t0.265006\t0.340000\t0.033000\n\t\n15:13:10.5\tlog_raw\tgps_raw\t#INSPVAXA,USB3,0,45.0,FINESTEERING,2107,281608.500,02000000,471d,15824;INS_ALIGNMENT_COMPLETE,INS_RTKFIXED,37.37125753147,126.72229922656,7.8853,22.3000,-0.0283,0.3023,-0.0044,-0.783072091,-0.564713007,90.330728689,0.4085,0.2746,0.5015,0.1092,0.0897,0.0746,0.1678,0.1684,5.1027,0f000001,0*a72eaeae\n\tsystem status\tnormal 2 28.100000 0 0\trobot status\t129.689481\t125.115817\t7.885300\t-0.783072\t-0.564713\t-0.330729\t0.279000\t-0.032000\n\t\n15:13:11.0\tlog_raw\tgps_raw\t#INSPVAXA,USB3,0,45.0,FINESTEERING,2107,281609.000,02000000,471d,15824;INS_ALIGNMENT_COMPLETE,INS_RTKFIXED,37.37125746019,126.72230086669,7.8844,22.3000,-0.0388,0.2946,-0.0124,-0.730333376,-0.851088036,90.998664332,0.4085,0.2746,0.5015,0.1092,0.0897,0.0746,0.1678,0.1684,5.1027,0f000001,0*4f9cf076\n\tsystem status\tnormal 2 28.100000 0 0\trobot status\t129.834761\t125.107904\t7.884400\t-0.730333\t-0.851088\t-0.998664\t0.221000\t-0.135000\n\t\n15:13:11.5\tlog_raw\tgps_raw\t#INSPVAXA,USB3,0,49.5,FINESTEERING,2107,281609.500,02000000,471d,15824;INS_ALIGNMENT_COMPLETE,INS_RTKFIXED,37.37125736767,126.72230251871,7.8837,22.3000,-0.0246,0.2829,-0.0110,-0.778570113,-1.137011227,91.636107067,0.4086,0.2746,0.5016,0.1092,0.0896,0.0746,0.1678,0.1683,5.1032,0f000001,0*f38f9db8\n\tsystem status\tnormal 2 28.100000 0 0\trobot status\t129.981095\t125.097633\t7.883700\t-0.778570\t-1.137011\t-1.636107\t0.440000\t0.190000\n\t\n15:13:12.0\tlog_raw\tgps_raw\t#INSPVAXA,USB3,0,49.5,FINESTEERING,2107,281610.000,02000000,471d,15824;INS_ALIGNMENT_COMPLETE,INS_RTKFIXED,37.37125727212,126.72230414457,7.8824,22.3000,-0.0153,0.2788,0.0009,-0.850299061,-1.150279108,92.167621233,0.4086,0.2746,0.5016,0.1092,0.0896,0.0746,0.1678,0.1683,5.1032,0f000001,0*9822d498\n\tsystem status\tnormal 2 28.100000 0 0\trobot status\t130.125111\t125.087026\t7.882400\t-0.850299\t-1.150279\t-2.167621\t0.336000\t0.036000\n\t\n15:13:12.5\tlog_raw\tgps_raw\t#DUALANTENNAHEADINGA,USB3,0,49.5,FINESTEERING,2107,281610.500,02000000,d426,15824;SOL_COMPUTED,L1_FLOAT,-1.000000000,84.036529541,-51.585266113,0.0,298.644531250,180.000000000,\"631T\",20,8,8,8,04,00,20,23*45ddee6b\n\tsystem status\tnormal 2 28.100000 0 0\trobot status\t130.267577\t125.074570\t7.879800\t-0.861795\t-1.127783\t-2.632731\t0.254000\t-0.079000\n\t\n15:13:13.0\tlog_raw\tgps_raw\t#DUALANTENNAHEADINGA,USB3,0,49.5,FINESTEERING,2107,281611.000,02000000,d426,15824;SOL_COMPUTED,L1_FLOAT,-1.000000000,84.902954102,-51.688964844,0.0,297.235992432,180.000000000,\"631T\",20,8,8,8,04,00,20,23*432775c3\n\tsystem status\tnormal 2 28.200000 0 0\trobot status\t130.408845\t125.061050\t7.877000\t-0.763463\t-1.049066\t-2.956519\t0.327000\t0.022000\n\t\n15:13:13.5\tlog_raw\tgps_raw\t#DUALANTENNAHEADINGA,USB3,0,48.0,FINESTEERING,2107,281611.500,02000000,d426,15824;SOL_COMPUTED,NARROW_FLOAT,-1.000000000,80.569839478,-43.681274414,0.0,202.652938843,180.000000000,\"631T\",19,9,9,7,04,00,20,23*350caf71\n\tsystem status\tnormal 2 28.200000 0 0\trobot status\t130.549816\t125.048476\t7.874600\t-0.783011\t-0.915067\t-3.207956\t0.305000\t-0.007000\n\t\n15:13:14.0\tlog_raw\tgps_raw\t#INSPVAXA,USB3,0,48.0,FINESTEERING,2107,281612.000,02000000,471d,15824;INS_ALIGNMENT_COMPLETE,INS_RTKFIXED,37.37125679959,126.72231051276,7.8723,22.3000,-0.0152,0.2724,0.0005,-0.625404023,-0.811400183,93.401020148,0.4082,0.2744,0.5017,0.1093,0.0896,0.0746,0.1677,0.1683,5.1044,0f000001,0*fa2c836e\n\tsystem status\tnormal 2 28.200000 0 0\trobot status\t130.689194\t125.034574\t7.872300\t-0.625404\t-0.811400\t-3.401020\t0.286000\t-0.007000\n\t\n15:13:14.5\tlog_raw\tgps_raw\t#INSPVAXA,USB3,0,46.0,FINESTEERING,2107,281612.500,02000000,471d,15824;INS_ALIGNMENT_COMPLETE,INS_RTKFIXED,37.37125664766,126.72231208737,7.8703,22.3000,-0.0138,0.2840,-0.0007,-0.548027474,-0.764885305,93.580702157,0.4082,0.2744,0.5017,0.1093,0.0896,0.0746,0.1677,0.1683,5.1050,0f000001,0*f22f9aa7\n\tsystem status\tnormal 2 28.200000 0 0\trobot status\t130.828671\t125.017710\t7.870300\t-0.548027\t-0.764885\t-3.580702\t0.303000\t0.001000\n\t\n15:13:15.0\tlog_raw\tgps_raw\t#INSPVAXA,USB3,0,46.0,FINESTEERING,2107,281613.000,02000000,471d,15824;INS_ALIGNMENT_COMPLETE,INS_RTKFIXED,37.37125650617,126.72231359099,7.8684,22.3000,-0.0180,0.2849,-0.0146,-0.566383475,-0.626492168,93.731901396,0.4082,0.2744,0.5017,0.1093,0.0896,0.0746,0.1677,0.1683,5.1050,0f000001,0*d3b26d7f\n\tsystem status\tnormal 2 28.200000 0 0\trobot status\t130.961859\t125.002005\t7.868400\t-0.566383\t-0.626492\t-3.731901\t0.302000\t0.017000\n\t\n15:13:15.5\tlog_raw\tgps_raw\t#DUALANTENNAHEADINGA,USB3,0,45.0,FINESTEERING,2107,281613.500,02000000,d426,15824;SOL_COMPUTED,L1_FLOAT,-1.000000000,83.088043213,-56.739044189,0.0,275.930023193,180.000000000,\"631T\",19,6,6,6,04,00,20,03*7fa5a20d\n\tsystem status\tnormal 2 28.200000 0 0\trobot status\t131.102518\t124.985371\t7.867300\t-0.590318\t-0.435554\t-3.801924\t0.298000\t0.013000\n\t\n15:13:16.0\tlog_raw\tgps_raw\t#DUALANTENNAHEADINGA,USB3,0,45.0,FINESTEERING,2107,281614.000,02000000,d426,15824;SOL_COMPUTED,L1_FLOAT,-1.000000000,82.710388184,-57.006988525,0.0,271.422698975,180.000000000,\"631T\",19,6,6,6,04,00,20,03*129b017c\n\tsystem status\tnormal 2 28.200000 0 0\trobot status\t131.247033\t124.968974\t7.866400\t-0.656975\t-0.282090\t-3.866351\t0.301000\t0.023000\n\t\n15:13:16.5\tlog_raw\tgps_raw\t#DUALANTENNAHEADINGA,USB3,0,46.5,FINESTEERING,2107,281614.500,02000000,d426,15824;SOL_COMPUTED,L1_FLOAT,-1.000000000,82.445899963,-51.127838135,0.0,347.003540039,180.000000000,\"631T\",19,6,6,6,04,00,20,03*63fc53d7\n\tsystem status\tnormal 2 28.200000 0 0\trobot status\t131.388610\t124.950539\t7.866200\t-0.618235\t-0.192706\t-3.884554\t0.288000\t0.035000\n\t\n15:13:17.0\tlog_raw\tgps_raw\t#DUALANTENNAHEADINGA,USB3,0,46.5,FINESTEERING,2107,281615.000,02000000,d426,15824;SOL_COMPUTED,L1_FLOAT,-1.000000000,81.371170044,-46.344207764,0.0,346.866485596,180.000000000,\"631T\",19,6,6,6,04,00,20,03*e0ade60f\n\tsystem status\tnormal 2 28.200000 0 0\trobot status\t131.535011\t124.930776\t7.867000\t-0.524107\t-0.062761\t-3.881484\t0.264000\t0.070000\n\t\n15:13:17.5\tlog_raw\tgps_raw\t#DUALANTENNAHEADINGA,USB3,0,50.5,FINESTEERING,2107,281615.500,02000000,d426,15824;SOL_COMPUTED,NARROW_FLOAT,-1.000000000,80.817100525,-47.001037598,0.0,207.681015015,180.000000000,\"631T\",20,6,6,6,04,00,20,03*9d84b137\n\tsystem status\tnormal 2 28.100000 0 0\trobot status\t131.678175\t124.911802\t7.867000\t-0.508048\t0.016781\t-3.694225\t0.301000\t0.012000\n\t\n15:13:18.0\tlog_raw\tgps_raw\t#DUALANTENNAHEADINGA,USB3,0,50.5,FINESTEERING,2107,281616.000,02000000,d426,15824;SOL_COMPUTED,NARROW_FLOAT,-1.000000000,81.509902954,-49.725524902,0.0,216.669723511,180.000000000,\"631T\",20,6,6,6,04,00,20,03*6356a6a7\n\tsystem status\tnormal 2 28.100000 0 0\trobot status\t131.819638\t124.894949\t7.867700\t-0.616373\t0.006653\t-3.292509\t0.272000\t0.063000\n\t\n15:13:18.5\tlog_raw\tgps_raw\t#INSPVAXA,USB3,0,47.5,FINESTEERING,2107,281616.500,02000000,471d,15824;INS_ALIGNMENT_COMPLETE,INS_RTKFIXED,37.37125540027,126.72232487564,7.8689,22.3000,-0.0235,0.2865,-0.0155,-0.776428369,-0.126871761,92.710705612,0.4096,0.2747,0.5015,0.1097,0.0898,0.0746,0.1674,0.1681,5.1098,0f000001,0*a35ee19b\n\tsystem status\tnormal 2 28.000000 0 0\trobot status\t131.961435\t124.879251\t7.868900\t-0.776428\t-0.126872\t-2.710706\t0.257000\t0.084000\n\t\n15:13:19.0\tlog_raw\tgps_raw\t#DUALANTENNAHEADINGA,USB3,0,47.5,FINESTEERING,2107,281617.000,02000000,d426,15824;SOL_COMPUTED,NARROW_FLOAT,-1.000000000,83.135253906,-45.598937988,0.0,198.452239990,180.000000000,\"631T\",19,7,7,6,04,00,20,03*722e59f8\n\tsystem status\tnormal 2 28.000000 0 0\trobot status\t132.100022\t124.865006\t7.870500\t-0.742883\t-0.197319\t-1.821921\t0.306000\t-0.010000\n\t\n15:13:19.5\tlog_raw\tgps_raw\t#INSPVAXA,USB3,0,49.0,FINESTEERING,2107,281617.500,02000000,471d,15824;INS_ALIGNMENT_COMPLETE,INS_RTKFIXED,37.37125515068,126.72232806022,7.8714,22.3000,-0.0152,0.2731,0.0045,-0.723483690,-0.404647650,90.811415851,0.4097,0.2748,0.5015,0.1095,0.0898,0.0746,0.1673,0.1681,5.1105,0f000001,0*086db8d4\n\tsystem status\tnormal 2 27.900000 0 0\trobot status\t132.243520\t124.851546\t7.871400\t-0.723484\t-0.404648\t-0.811416\t0.289000\t0.038000\n\t\n15:13:20.0\tlog_raw\tgps_raw\t#INSPVAXA,USB3,0,49.0,FINESTEERING,2107,281618.000,02000000,471d,15824;INS_ALIGNMENT_COMPLETE,INS_RTKFIXED,37.37125505743,126.72232965261,7.8715,22.3000,-0.0112,0.2768,-0.0033,-0.719605917,-0.592487460,89.836730545,0.4097,0.2748,0.5015,0.1095,0.0898,0.0746,0.1673,0.1681,5.1105,0f000001,0*7f7a4829\n\tsystem status\tnormal 2 27.900000 0 0\trobot status\t132.384571\t124.841194\t7.871500\t-0.719606\t-0.592487\t0.163269\t0.292000\t0.035000\n\t\n15:13:20.5\tlog_raw\tgps_raw\t#DUALANTENNAHEADINGA,USB3,0,49.5,FINESTEERING,2107,281618.500,
